vi "Getting Started with Attributes.vi"() -> ()   [LabVIEW 2023]
doc: "The Getting Started with Attributes example introduces the user to programmatically interacting with camera attributes."
uses:
  <vilib>/vision/driver/IMAQdx.llb/IMAQdx Attribute Type.ctl
  <vilib>/vision/driver/NI_Vision_Acquisition_Software.lvlib
  <resource>/objmgr/imaqdx.rc
panel:
  in  "Stop":bool
  out "Active Attribute Details":string
  in  "Active Attribute":u16(ring) caption="Active Attribute (Index:       )" items=["AcquisitionAttributes::Bayer::Algorithm", "AcquisitionAttributes::Bayer::GainB", "AcquisitionAttributes::Bayer::GainG", "AcquisitionAttributes::Bayer::GainR", "AcquisitionAttributes::Bayer::Pattern", "CameraAttributes::AcquisitionControls::AcquisitionFrameRateAbs", "CameraAttributes::AcquisitionControls::TriggerMode", "CameraAttributes::AcquisitionControls::TriggerSelector", "CameraAttributes::AcquisitionControls::TriggerSoftware", "CameraAttributes::AcquisitionControls::TriggerSource", "CameraAttributes::AnalogControls::GainAbs", "CameraAttributes::AnalogControls::GainSelector", "CameraAttributes::ImageSizeControls::Height", "CameraAttributes::ImageSizeControls::PayloadSize", "CameraAttributes::ImageSizeControls::PixelFormat", "CameraAttributes::ImageSizeControls::TestImageSelector", "CameraAttributes::ImageSizeControls::Width", "AcquisitionAttributes::BitsPerPixel", "AcquisitionAttributes::HardwareMaximumQueuedBufferCount", "AcquisitionAttributes::HardwareRequeueBufferListThreshold", "AcquisitionAttributes::ImageDecoderCopyMode", "AcquisitionAttributes::OutputImageType", "AcquisitionAttributes::OverwriteMode", "AcquisitionAttributes::ReceiveTimestampMode", "AcquisitionAttributes::ShiftPixelBits", "AcquisitionAttributes::SwapPixelBytes", "AcquisitionAttributes::Timeout", "CameraInformation::BaseAddress", "CameraInformation::BusType", "CameraInformation::ModelName", "CameraInformation::SerialNumberHigh", "CameraInformation::SerialNumberLow", "CameraInformation::VendorName", "StatusInformation::AcqInProgress", "StatusInformation::LastBufferCount", "StatusInformation::LastBufferNumber", "StatusInformation::LostBufferCount"]
  out "Number of Attributes":i32
  out "Initial Attribute Settings":T2(array[cluster])
  in  "Show Only Camera Attributes":bool
  in  "Visibility":enum16{"Simple", "Intermediate", "Advanced"}(ring)=enum."Advanced"
  in  "Camera Name":refnum<k21> caption="IMAQdx Session"
  # "Overview: Demonstrates how to enumerate camera attributes and view detailed settings for each attribute.\nRequirements: Vision Acquisition Software\nInstructions: \n1. Select the Camera Name\n2. Set the Visibility and Show Only Camera Attributes as desired. Read more about these options in the notes on the Block Diagram.\n2. Run the VI"
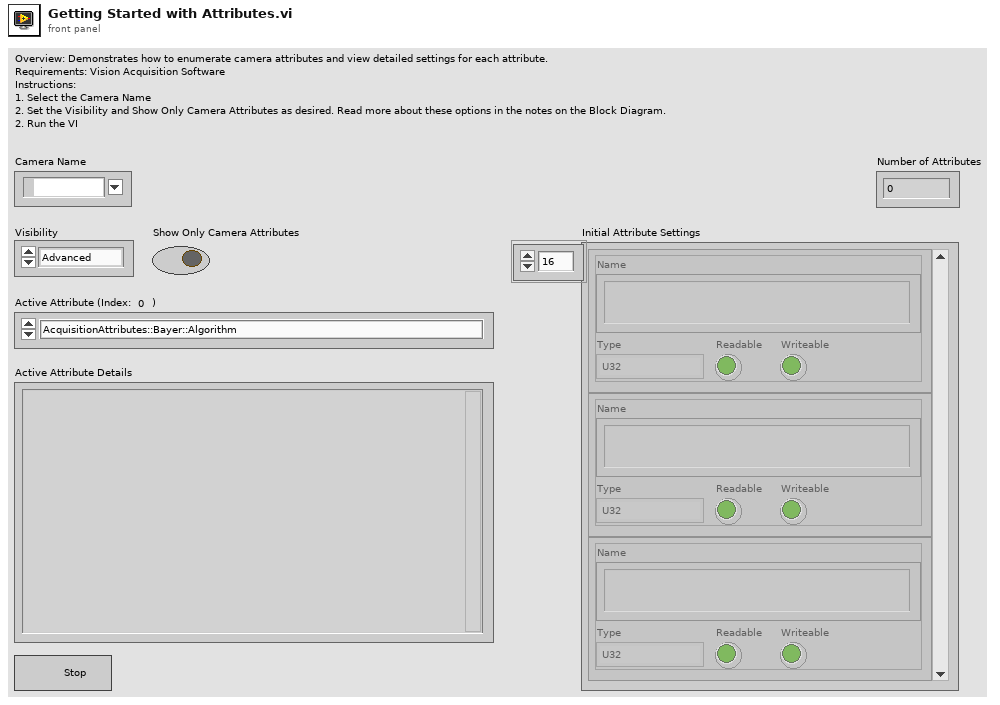
[diagram p1: front panel]
types:
  T1 = typedef "NI_Vision_Acquisition_Software.lvlib/IMAQdx Attribute Type.ctl" = enum32{"U32", "I64", "DBL", "String", "Enum", "Bool", "Command"}
  T2 = cluster{"Type":T1, "Readable":bool, "Writeable":bool, "Name":string}[]
  T3 = typedef "IMAQdx.ctl" = refnum<k21>
  T4 = cluster{"Attribute Type":T1, "Readable":bool, "Writable":bool, "Attribute Name":string}[]
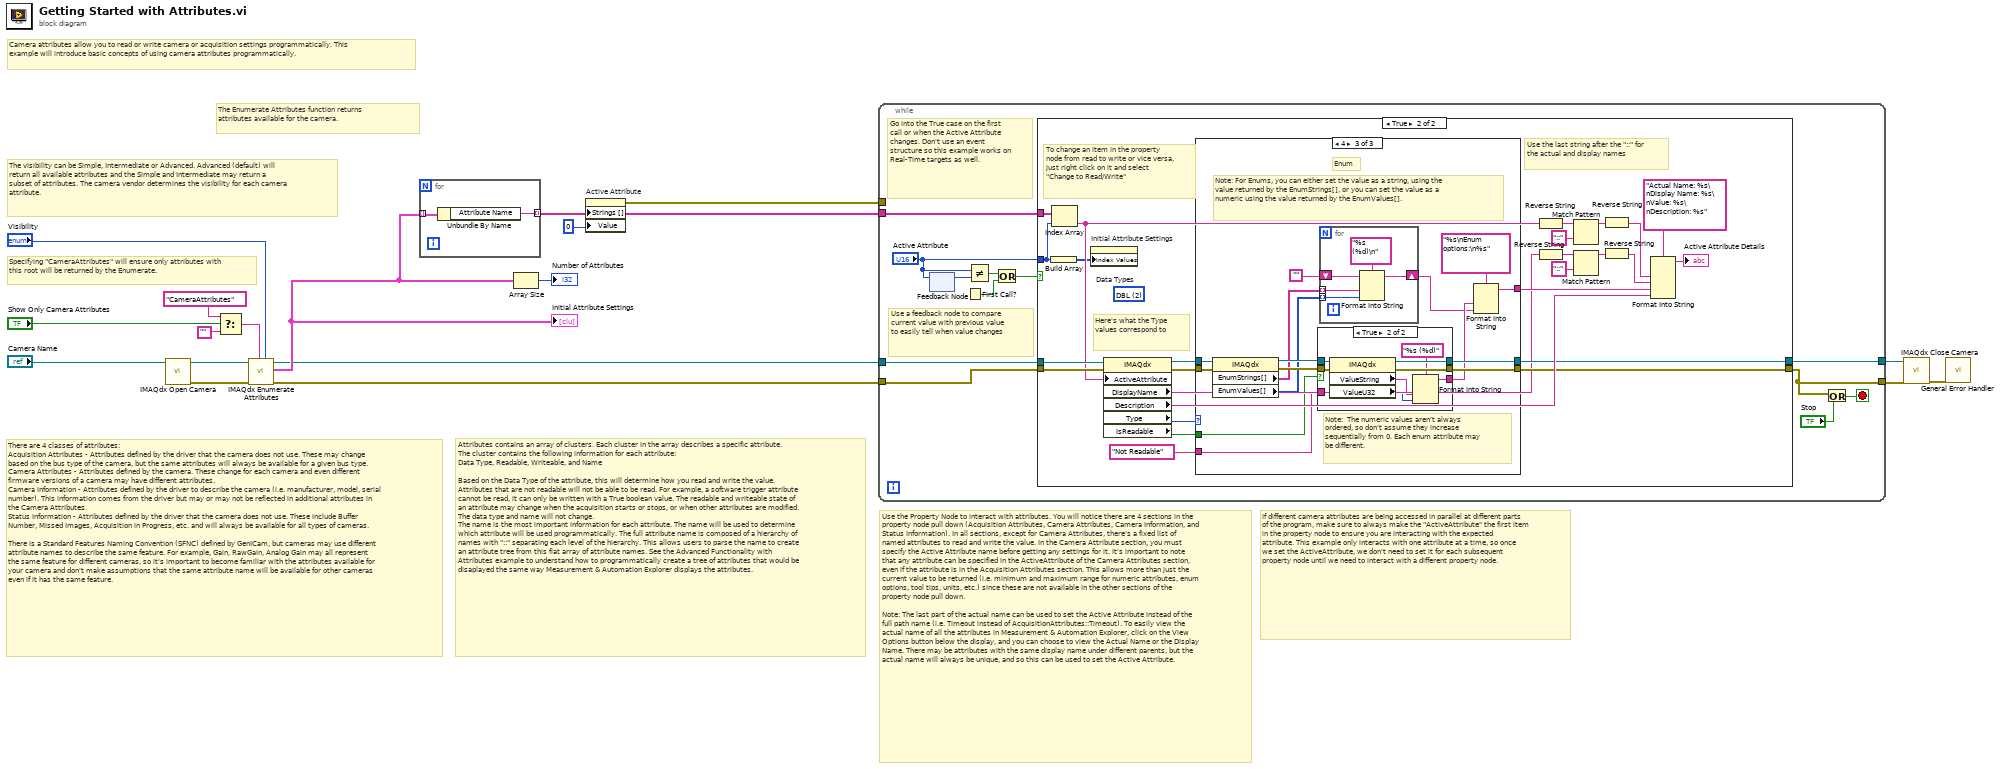
[diagram p0: block diagram]
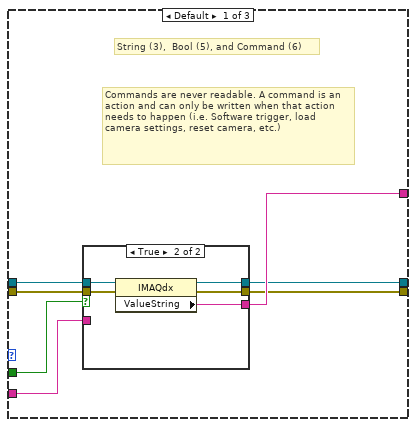
[diagram p3: hidden frame]
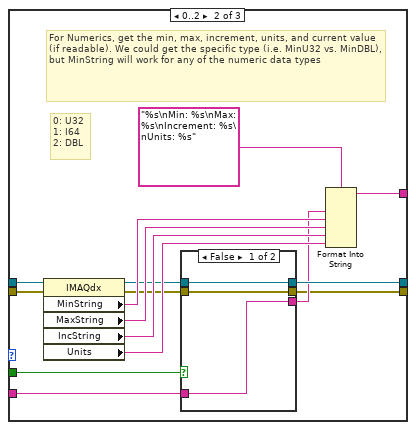
[diagram p5: hidden frame]
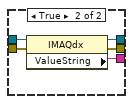
[diagram p6: hidden frame]
diagram:
  # "If different camera attributes are being accessed in parallel at different parts of the program, make sure to always make the \"ActiveAttribute\" the first item in the property node to ensure you are interacting with the expected attribute. This example only interacts with one attribute at a time, so once we set the ActiveAttribute, we don't need to set it for each subsequent property node until we need to interact with a different property node."
  # "Use the Property Node to interact with attributes. You will notice there are 4 sections in the property node pull down (Acquisition Attributes, Camera Attributes, Camera Information, and Status Information). In all sections, except for Camera Attributes, there's a fixed list of named attributes to read and write the value. In the Camera Attribute section, you must specify the Active Attribute name before getting any settings for it. It's important to note that any attribute can be specified in the ActiveAttribute of the Camera Attributes section, even if the attribute is in the Acquisition Attributes section. This allows more than just the current value to be returned (i.e. minimum and maximum range for numeric attributes, enum options, tool tips, units, etc.) since these are not available in the other sections of the property node pull down.\n\nNote: The last part of the actual name can be used to set the Active Attribute instead of the full path name (i.e. Timeout instead of AcquisitionAttributes::Timeout). To easily view the actual name of all the attributes in Measurement & Automation Explorer, click on the View Options button below the display, and you can choose to view the Actual Name or the Display Name. There may be attributes with the same display name under different parents, but the actual name will always be unique, and so this can be used to set the Active Attribute."
  # "Specifying \"CameraAttributes\" will ensure only attributes with this root will be returned by the Enumerate."
  # "Attributes contains an array of clusters. Each cluster in the array describes a specific attribute. \nThe cluster contains the following information for each attribute:\nData Type, Readable, Writeable, and Name \n\nBased on the Data Type of the attribute, this will determine how you read and write the value.\nAttributes that are not readable will not be able to be read. For example, a software trigger attribute cannot be read, it can only be written with a True boolean value. The readable and writeable state of an attribute may change when the acquisition starts or stops, or when other attributes are modified. The data type and name will not change.\nThe name is the most important information for each attribute. The name will be used to determine which attribute will be used programmatically. The full attribute name is composed of a hierarchy of names with \"::\" separating each level of the hierarchy. This allows users to parse the name to create an attribute tree from this flat array of attribute names. See the Advanced Functionality with Attributes example to understand how to programmatically create a tree of attributes that would be disaplayed the same way Measurement & Automation Explorer displays the attributes."
  # "There are 4 classes of attributes:\nAcquisition Attributes - Attributes defined by the driver that the camera does not use. These may change based on the bus type of the camera, but the same attributes will always be available for a given bus type.\nCamera Attributes - Attributes defined by the camera. These change for each camera and even different firmware versions of a camera may have different attributes.\nCamera Information - Attributes defined by the driver to describe the camera (i.e. manufacturer, model, serial number). This information comes from the driver but may or may not be reflected in additional attributes in the Camera Attributes.\nStatus Information - Attributes defined by the driver that the camera does not use. These include Buffer Number, Missed Images, Acquisition in Progress, etc. and will always be available for all types of cameras.\n\nThere is a Standard Features Naming Convention (SFNC) defined by GenICam, but cameras may use different attribute names to describe the same feature. For example, Gain, RawGain, Analog Gain may all represent the same feature for different cameras, so it's important to become familiar with the attributes available for your camera and don't make assumptions that the same attribute name will be available for other cameras even if it has the same feature."
  # "Camera attributes allow you to read or write camera or acquisition settings programmatically. This example will introduce basic concepts of using camera attributes programmatically."
  # "The visibility can be Simple, Intermediate or Advanced. Advanced (default) will return all available attributes and the Simple and Intermediate may return a subset of attributes. The camera vendor determines the visibility for each camera attribute."
  # "The Enumerate Attributes function returns attributes available for the camera."
  n1 = call <vilib>:"IMAQdx Open Camera.vi"("Session In"="Camera Name") -> ("error out"=w16:errorcluster, "Session Out"=w15:T3)  [unwired: 2 in, 7 out]
  n2 = Select(t="CameraAttributes", s="Show Only Camera Attributes", f="") -> (s? t:f=w12:string)
  n3 = call <vilib>:"IMAQdx Enumerate Attributes.vi"("Visibility"="Visibility", "Root"=w12, "error in"=w16, "Session In"=w15) -> ("error out"=w5:errorcluster, "Attribute Information Array"=w8:T4, "Session Out"=w7:T3)  [unwired: 5 out]
  "Initial Attribute Settings" <- w8
  n4 = for {
    tunnel: w8 -> [w20] mode=indexing
    tunnel: [w19] -> w4 mode=indexing
    n5 = Unbundle By Name(w20) -> ("Attribute Name"=w19:string)
  }
  n6 = Array Size(array=w8) -> (size(s)=→"Number of Attributes":i32)
  n7 = property on="Active Attribute" class="Ring (strict)"("Strings []"=w4, "Value"=0) -> (error out=w6:errorcluster)  [unwired: 2 in, 1 out]
  n8 = while {
    tunnel: w7 -> [w26]
    tunnel: w6 -> [_]
    tunnel: w5 -> [w25]
    tunnel: w4 -> [w32]
    tunnel: [w23] -> w3
    tunnel: [w22] -> w2
    stop <- w21 stop-if-true
    # "Use a feedback node to compare current value with previous value to easily tell when value changes"
    # "Go into the True case on the first call or when the Active Attribute changes. Don't use an event structure so this example works on Real-Time targets as well."
    n9 = feedback-in #1("Active Attribute") -> ()
    n10 = feedback #1() -> (w31:u16)  [unwired: 1 in]
    n11 = First Call?() -> (First Call?: T/F=w29:bool)
    n12 = Not Equal?(x="Active Attribute", y=w31) -> (x != y?=w30:bool)
    n13 = Or(x=w30, y=w29) -> (x .or. y?=w28:bool)
    n14 = case shown="True" w28 {
      tunnel: w32 -> [_ w60]
      tunnel: "Active Attribute" -> [_ w36]
      tunnel: w26 -> [w34 w59]
      tunnel: w25 -> [w33 w58]
      tunnel: [w34 w48] -> w23
      tunnel: [w33 w47] -> w22
      frame False {
        # "Nothing changed."
      }
      frame True {
        (unwired) u32 2 items=["U32", "I64", "DBL", "String", "Enum", "Bool", "Command"]  # Data Types
        # "Here's what the Type values correspond to"
        # "Use the last string after the \"::\" for the actual and display names"
        # "To change an item in the property node from read to write or vice versa, just right click on it and select \"Change to Read/Write\""
        n15 = Build Array(w36) -> (w35:u16[])
        n16 = Index Array(array=w60, index=w36) -> (element=w43:string)
        n17 = property on="Initial Attribute Settings" class="Arr (strict)"("Index Values"=w35) -> ()  [unwired: 2 in, 2 out]
        n18 = property class="IMAQdx"(reference=w59, error in=w58, "ActiveAttribute"=w43) -> (reference out=w57:T3, error out=w56:errorcluster, "DisplayName"=w38:string, "Description"=w52:string, "Type"=w55:u32, "IsReadable"=w50:bool)
        n19 = case shown="4" w55 {
          tunnel: w57 -> [w67 w90 w106]
          tunnel: w56 -> [w66 w89 w105]
          tunnel: [w64 w83 w107] -> w51
          tunnel: w50 -> [w65 w82 w113]
          tunnel: "Not Readable" ("ValueString") -> [w61 w79 w110]
          tunnel: [w63 w78 w112] -> w48
          tunnel: [w62 w76 w111] -> w47
          frame Default {
            # "Commands are never readable. A command is an action and can only be written when that action needs to happen (i.e. Software trigger, load camera settings, reset camera, etc.)"
            # "String (3),  Bool (5), and Command (6)"
            n20 = case shown="True" w65 {
              tunnel: w67 -> [w70 w75]
              tunnel: w66 -> [w69 w74]
              tunnel: [w68 w73] -> w64
              tunnel: [w70 w72] -> w63
              tunnel: [w69 w71] -> w62
              tunnel: w61 -> [w68 _]
              frame False {
              }
              frame True {
                n21 = property class="IMAQdx"(reference=w75, error in=w74) -> (reference out=w72:T3, error out=w71:errorcluster, "ValueString"=w73:string)
              }
            }
          }
          frame 0..2 {
            # "For Numerics, get the min, max, increment, units, and current value (if readable). We could get the specific type (i.e. MinU32 vs. MinDBL), but MinString will work for any of the numeric data types"
            # "0: U32\n1: I64\n2: DBL"
            n22 = property class="IMAQdx"(reference=w90, error in=w89) -> (reference out=w81:T3, error out=w80:errorcluster, "MinString"=w87:string, "MaxString"=w86:string, "IncString"=w85:string, "Units"=w84:string)
            n23 = case shown="False" w82 {
              tunnel: w81 -> [w92 w97]
              tunnel: w80 -> [w91 w96]
              tunnel: [w93 w98] -> w77
              tunnel: w79 -> [w93 _]
              tunnel: [w92 w95] -> w78
              tunnel: [w91 w94] -> w76
              frame False {
              }
              frame True {
                n24 = property class="IMAQdx"(reference=w97, error in=w96) -> (reference out=w95:T3, error out=w94:errorcluster, "ValueString"=w98:string)
              }
            }
            n25 = Format Into String(format string="%s\nMin: %s\nMax: %s\nIncrement: %s\nUnits: %s", w77, w87, w86, w85, w84) -> (resulting string=w83:string)  [unwired: 2 in, 1 out]
          }
          frame 4 {
            # "Note:  The numeric values aren't always ordered, so don't assume they increase sequentially from 0. Each enum attribute may be different."
            # "Note: For Enums, you can either set the value as a string, using the value returned by the EnumStrings[], or you can set the value as a numeric using the value returned by the EnumValues[]."
            # "Enum"
            n26 = property class="IMAQdx"(reference=w106, error in=w105) -> (reference out=w104:T3, error out=w103:errorcluster, "EnumStrings[]"=w102:string[], "EnumValues[]"=w101:u32[])
            n27 = case shown="True" w113 {
              tunnel: w104 -> [w121 w129]
              tunnel: w103 -> [w120 w128]
              tunnel: [w119 w124] -> w108
              tunnel: [w121 w127] -> w112
              tunnel: [w120 w126] -> w111
              tunnel: w110 -> [w119 _]
              frame False {
              }
              frame True {
                n28 = property class="IMAQdx"(reference=w129, error in=w128) -> (reference out=w127:T3, error out=w126:errorcluster, "ValueString"=w123:string, "ValueU32"=w125:u32)
                n29 = Format Into String(format string="%s (%d)", w123, w125) -> (resulting string=w124:string)  [unwired: 2 in, 1 out]
              }
            }
            n30 = for {
              tunnel: w102 -> [w116] mode=indexing
              tunnel: w101 -> [w115] mode=indexing
              shift-right: [w114] -> w99
              shift-left: "" -> [w118]
              n31 = Format Into String(format string="%s (%d)\n", initial string=w118, w116, w115) -> (resulting string=w114:string)  [unwired: 1 in, 1 out]
            }
            n32 = Format Into String(format string="%s\nEnum options:\n%s", w108, w99) -> (resulting string=w107:string)  [unwired: 2 in, 1 out]
          }
        }
        n33 = Reverse String(1:w43) -> (0:w46:string)
        n34 = Reverse String(1:w38) -> (0:w39:string)
        n35 = Match Pattern(string=w46, regular expression="::") -> (before substring=w44:string)  [unwired: 1 in, 3 out]
        n36 = Match Pattern(string=w39, regular expression="::") -> (before substring=w41:string)  [unwired: 1 in, 3 out]
        n37 = Reverse String(1:w44) -> (0:w42:string)
        n38 = Reverse String(1:w41) -> (0:w37:string)
        n39 = Format Into String(format string="Actual Name: %s\nDisplay Name: %s\nValue: %s\nDescription: %s", w42, w37, w51, w52) -> (resulting string=→"Active Attribute Details":string)  [unwired: 2 in, 1 out]
      }
    }
    n40 = Or(x=w22, y="Stop") -> (x .or. y?=w21:bool)
  }
  n41 = call <vilib>:"IMAQdx Close Camera.vi"("error in"=w2, "Session In"=w3) -> ("error out"=w10:errorcluster)  [unwired: 9 out]
  n42 = call <vilib>:"General Error Handler.vi"("error in (no error)"=w10) -> ()  [unwired: 2 in, 13 out]
